vi "CRISPR Program.vi"() -> ()   [LabVIEW 2024]
uses:
  States Enum.ctl
panel:
  in  "Splice 1: Base Pair to be used":enum16{"T-A", "A-T", "C-G", "G-C"}(ring)
  in  "Splice 1: Base Pair No.  in Codon":dbl=1.0 min=1.0 max=3.0
  in  "Splice 1: Codon No.":dbl=1.0 min=1.0 max=5.0
  out "% of C-G(G-C) in Modified DNA Sequence":dbl format="%#.0f"
  out "% of A-T(T-A) in Modified DNA Sequence":dbl format="%#.0f"
  out "Modified DNA A-COUNT":i32
  out "Modified DNA C-COUNT":i32
  out "Modified DNA G-COUNT":i32
  out "Modified DNA T-COUNT":i32
  in  "Stop":bool
  out "Modified DNA Sequence":string[][](array[string])
  in  "Splice":bool
  in  "DNA Splice Selector":T1(ring)=enum."Splice 2"
  out "% of C-G(G-C) in DNA Sequence":dbl format="%#.0f"
  out "% of A-T(T-A) in DNA Sequence":dbl format="%#.0f"
  out "DNA A-COUNT":i32
  out "DNA C-COUNT":i32
  out "DNA G-COUNT":i32
  out "DNA T-COUNT":i32
  out "DNA Sequence":string[][](array[string])
  out "RNA Sequence with Mutation Genes Removed":string[][](array[string])
  out "error out":errorcluster
  in  "error in (no error)":errorcluster
  out "Original RNA Sequence":string[][](array[string])
  # "Normal DNA Sequence"
  # "Modified DNA Sequence"
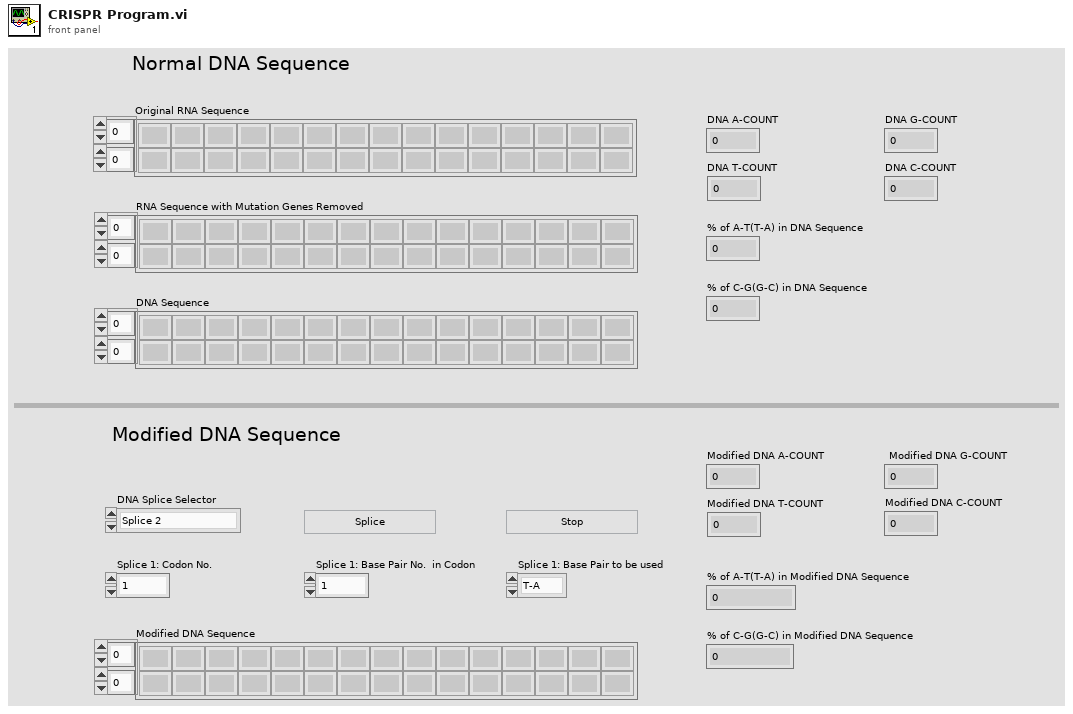
[diagram p1: front panel]
types:
  T1 = enum16{"Splice 1", "Splice 2", "Splice 3", "Splice 4", "No Splice"}
  T2 = typedef "States Enum.ctl" = enum16{"Remove Mutation", "Initialize", "DNA Sequence", "DNA Result", "Modified DNA Sequence", "Modified DNA Result", "Wait"}
  T3 = enum8{"Enabled", "Disabled", "Disabled and Grayed Out"}
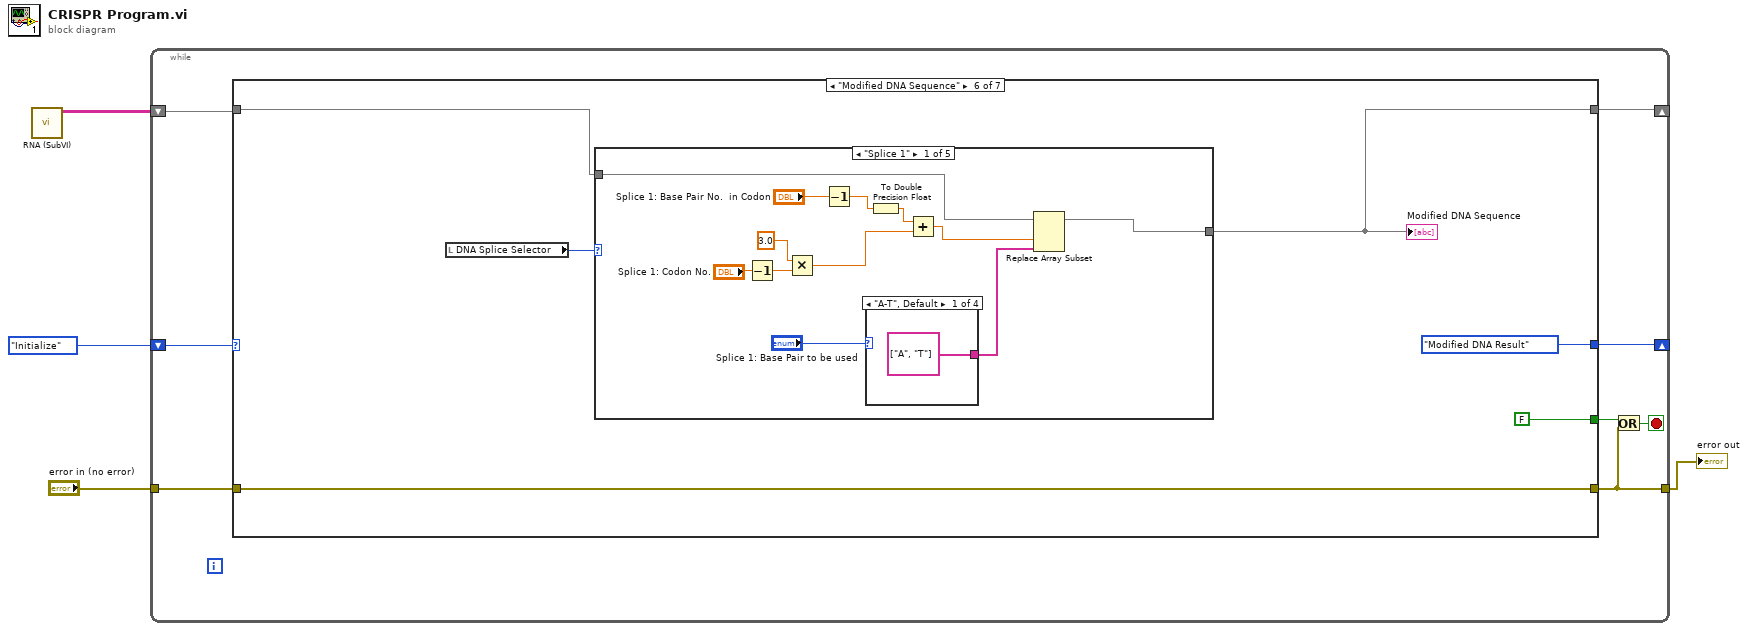
[diagram p0: block diagram]
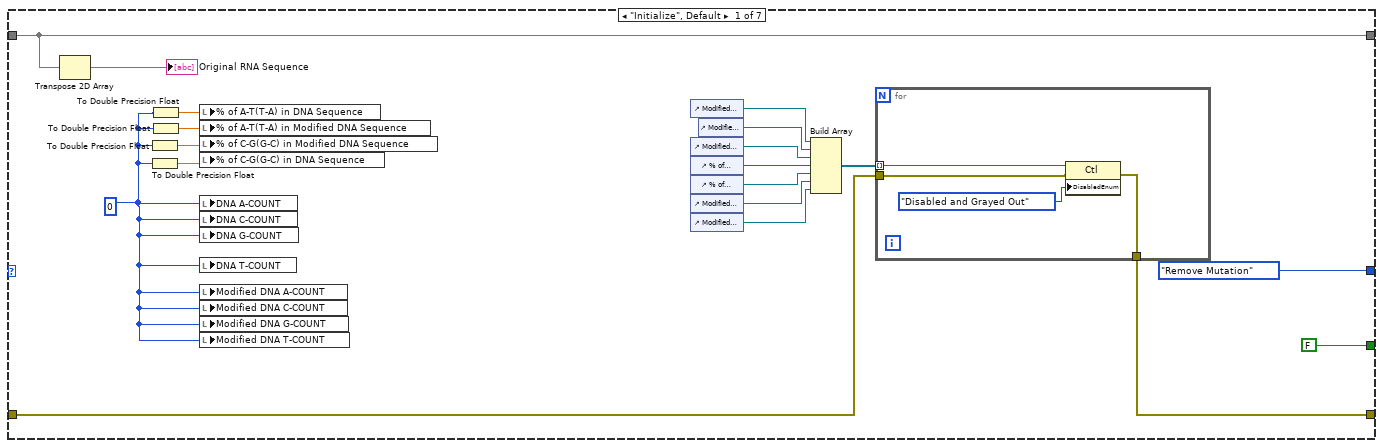
[diagram p2: hidden frame]
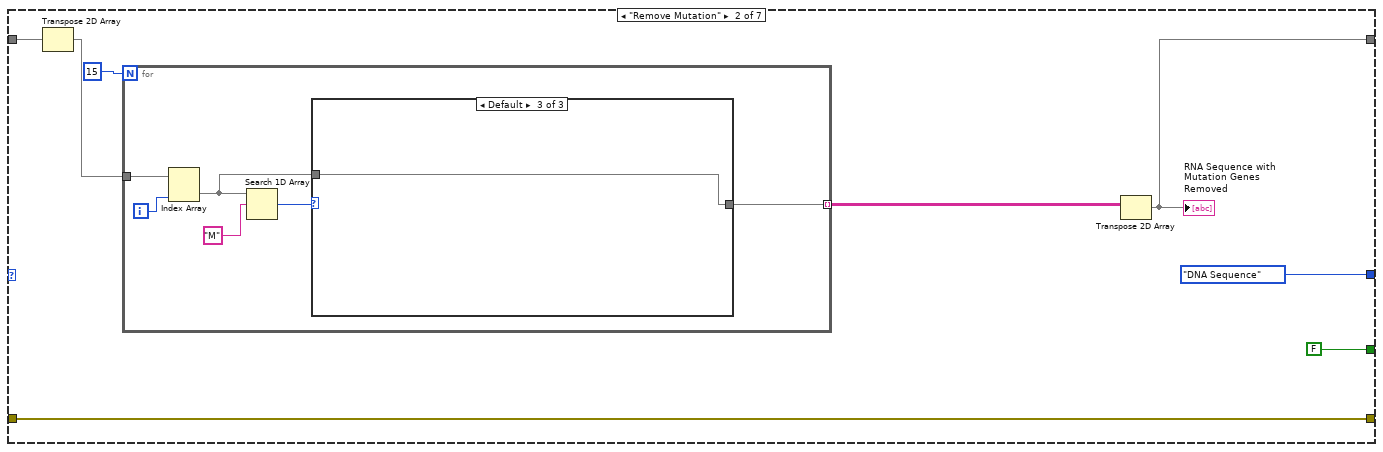
[diagram p3: hidden frame]
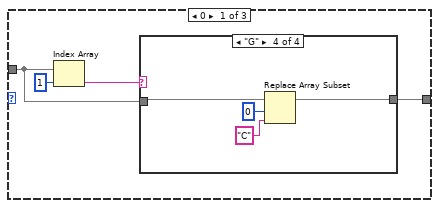
[diagram p4: hidden frame]
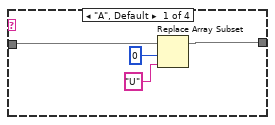
[diagram p5: hidden frame]
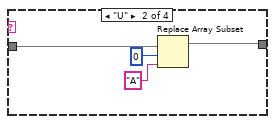
[diagram p6: hidden frame]
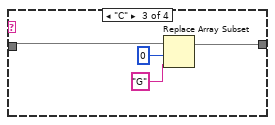
[diagram p7: hidden frame]
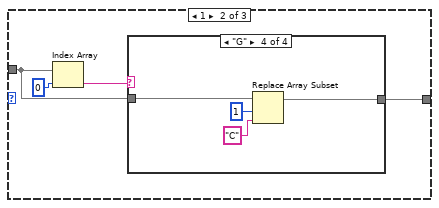
[diagram p8: hidden frame]
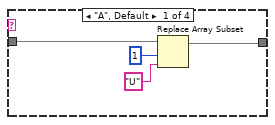
[diagram p9: hidden frame]
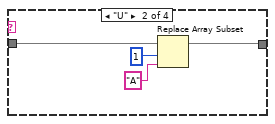
[diagram p10: hidden frame]
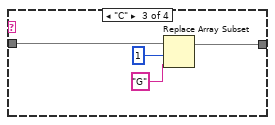
[diagram p11: hidden frame]
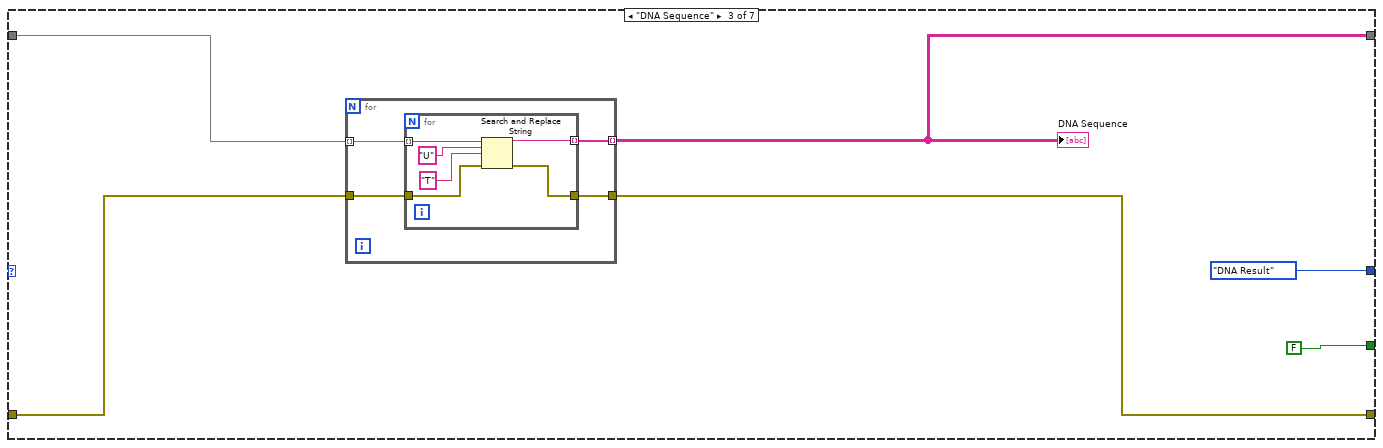
[diagram p12: hidden frame]
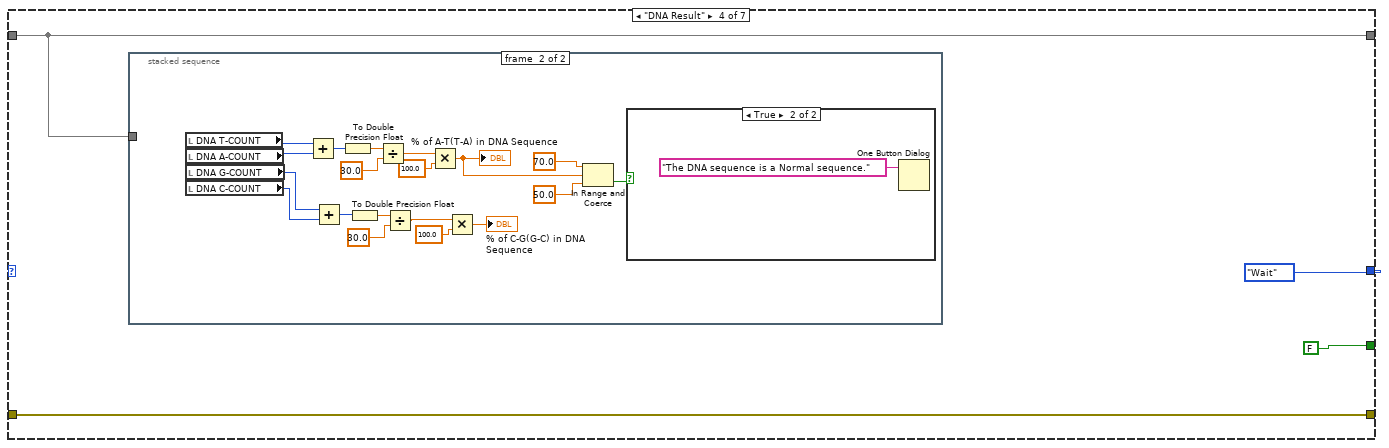
[diagram p13: hidden frame]
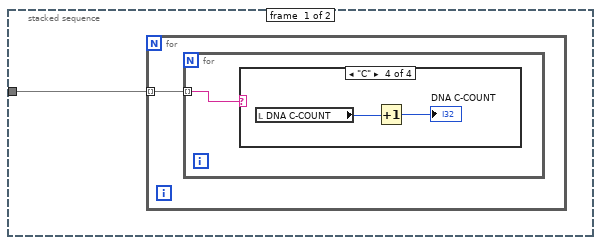
[diagram p14: hidden frame]
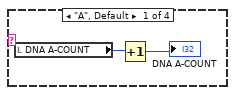
[diagram p15: hidden frame]
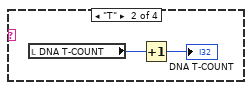
[diagram p16: hidden frame]
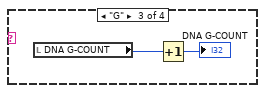
[diagram p17: hidden frame]
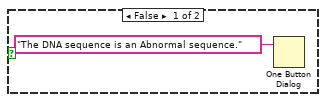
[diagram p18: hidden frame]
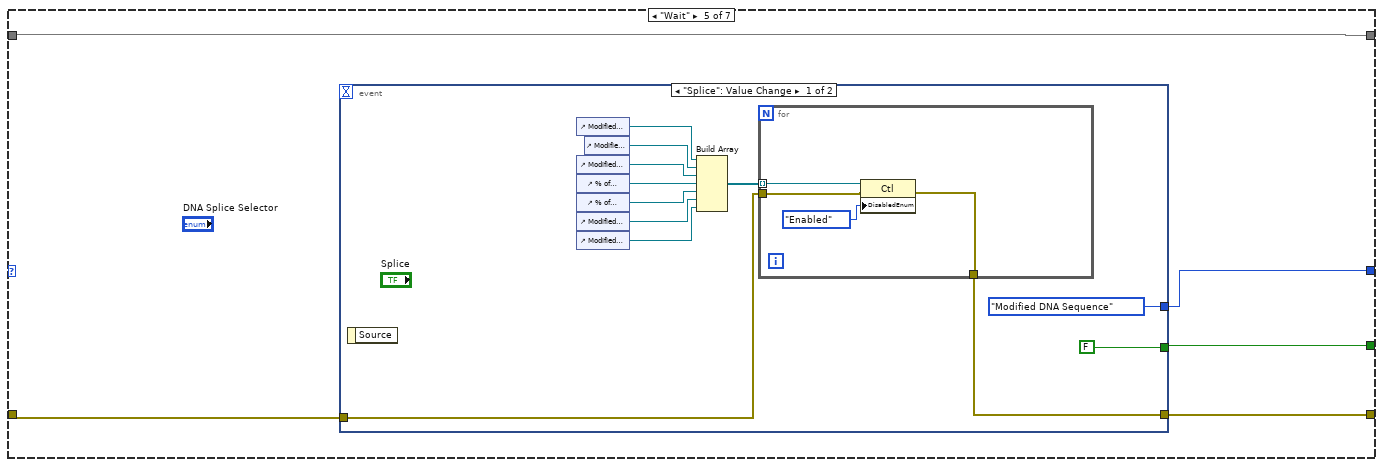
[diagram p19: hidden frame]
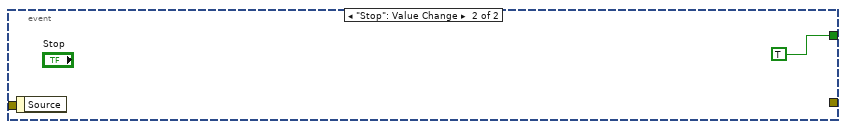
[diagram p20: hidden frame]
diagram:
  n1 = call "RNA (SubVI).vi"() -> ("RNA Sequence"=w2:string[][])  [unwired: 11 in]
  n2 = while {
    shift-right: [w5] -> _
    shift-left: States_Enum."Initialize" -> [w6]
    shift-right: [w11] -> _
    shift-left: w2 -> [w12]
    tunnel: "error in (no error)" -> [w10]
    tunnel: [w7] -> w3
    stop <- w9 stop-if-true
    n3 = case shown="\"Modified DNA Sequence\"" w6 {
      tunnel: w12 -> [w30 w43 w96 w109 w147 w167 w217]
      tunnel: [w30 w37 w95 w109 w147 w165 w217] -> w11
      tunnel: [States_Enum."Remove Mutation" States_Enum."DNA Sequence" States_Enum."DNA Result" States_Enum."Wait" w145 States_Enum."Modified DNA Result" States_Enum."Initialize"] -> w5
      tunnel: w10 -> [w14 w41 w93 w110 w146 w170 w218]
      tunnel: [w13 w41 w92 w110 w143 w170 w218] -> w7
      tunnel: [FALSE FALSE FALSE FALSE w144 FALSE TRUE] -> w8
      frame "Initialize", Default {
        w23 = 0 ("DNA A-COUNT")
        n4 = Transpose 2D Array(2D array=w30) -> (transposed array=→"Original RNA Sequence":string[][])
        n5 = To Double Precision Float(number=w23) -> (double precision float=w25:dbl)
        n6 = To Double Precision Float(number=w23) -> (double precision float=w24:dbl)
        n7 = To Double Precision Float(number=w23) -> (double precision float=w27:dbl)
        n8 = To Double Precision Float(number=w23) -> (double precision float=w26:dbl)
        n9 = local write "% of A-T(T-A) in DNA Sequence"(w27) -> ()
        n10 = local write "% of A-T(T-A) in Modified DNA Sequence"(w26) -> ()
        n11 = local write "% of C-G(G-C) in Modified DNA Sequence"(w25) -> ()
        n12 = local write "% of C-G(G-C) in DNA Sequence"(w24) -> ()
        n13 = local write "DNA A-COUNT"(w23) -> ()
        n14 = local write "DNA C-COUNT"(w23) -> ()
        n15 = local write "DNA G-COUNT"(w23) -> ()
        n16 = local write "DNA T-COUNT"(w23) -> ()
        n17 = local write "Modified DNA A-COUNT"(w23) -> ()
        n18 = local write "Modified DNA C-COUNT"(w23) -> ()
        n19 = local write "Modified DNA G-COUNT"(w23) -> ()
        n20 = local write "Modified DNA T-COUNT"(w23) -> ()
        n21 = control-ref of="Modified DNA C-COUNT"() -> (w22:refnum<vi>)
        n22 = control-ref of="Modified DNA A-COUNT"() -> (w20:refnum<vi>)
        n23 = control-ref of="% of C-G(G-C) in Modified DNA Sequence"() -> (w19:refnum<vi>)
        n24 = control-ref of="% of A-T(T-A) in Modified DNA Sequence"() -> (w18:refnum<vi>)
        n25 = control-ref of="Modified DNA T-COUNT"() -> (w17:refnum<vi>)
        n26 = control-ref of="Modified DNA G-COUNT"() -> (w16:refnum<vi>)
        n27 = control-ref of="Modified DNA Sequence"() -> (w21:refnum<vi>)
        n28 = Build Array(w22, w21, w20, w19, w18, w17, w16) -> (w15:refnum<vi>[])
        n29 = for {
          tunnel: w15 -> [w35] mode=indexing
          tunnel: w14 -> [w33]
          tunnel: [w32] -> w13
          n30 = property class="Ctl"(reference=w35, error in=w33, "DisabledEnum"=T3."Disabled and Grayed Out" ("Disabled")) -> (error out=w32:errorcluster)  [unwired: 1 out]
        }
      }
      frame "Remove Mutation" {
        n31 = Transpose 2D Array(2D array=w43) -> (transposed array=w39:string[][])
        n32 = for {
          N: 15 -> [_]
          tunnel: [w47] -> w38 mode=indexing
          tunnel: w39 -> [w46]
          i -> [w49]
          n33 = Index Array(array=w46, index (col)=w49) -> (element=w45:string[])  [unwired: 1 in]
          n34 = Search 1D Array(1D array=w45, element="M") -> (index of element=w48:i32)  [unwired: 1 in]
          n35 = case shown="Default" w48 {
            tunnel: w45 -> [w51 w71 w90]
            tunnel: [w52 w72 w90] -> w47
            frame 0 {
              n36 = Index Array(array=w51, index=1) -> (element=w50:string)
              n37 = case shown="\"G\"" w50 {
                tunnel: w51 -> [w54 w58 w62 w66]
                tunnel: [w55 w59 w63 w67] -> w52
                frame "A", Default {
                  n38 = Replace Array Subset(array=w54, new element="U" ("element"), index=0) -> (w55:string[])
                }
                frame "U" {
                  n39 = Replace Array Subset(array=w58, new element="A" ("element"), index=0) -> (w59:string[])
                }
                frame "C" {
                  n40 = Replace Array Subset(array=w62, new element="G" ("element"), index=0) -> (w63:string[])
                }
                frame "G" {
                  n41 = Replace Array Subset(array=w66, new element="C" ("element"), index=0) -> (w67:string[])
                }
              }
            }
            frame 1 {
              n42 = Index Array(array=w71, index=0) -> (element=w70:string)
              n43 = case shown="\"G\"" w70 {
                tunnel: w71 -> [w74 w78 w82 w86]
                tunnel: [w75 w79 w83 w87] -> w72
                frame "A", Default {
                  n44 = Replace Array Subset(array=w74, new element="U" ("element"), index=1) -> (w75:string[])
                }
                frame "U" {
                  n45 = Replace Array Subset(array=w78, new element="A" ("element"), index=1) -> (w79:string[])
                }
                frame "C" {
                  n46 = Replace Array Subset(array=w82, new element="G" ("element"), index=1) -> (w83:string[])
                }
                frame "G" {
                  n47 = Replace Array Subset(array=w86, new element="C" ("element"), index=1) -> (w87:string[])
                }
              }
            }
            frame Default {
            }
          }
        }
        n48 = Transpose 2D Array(2D array=w38) -> (transposed array=w37:string[][])
        "RNA Sequence with Mutation Genes Removed" <- w37
      }
      frame "DNA Sequence" {
        n49 = for {
          tunnel: w96 -> [w100] mode=indexing
          tunnel: [w99] -> w95 mode=indexing
          tunnel: w93 -> [w98]
          tunnel: [w97] -> w92
          n50 = for {
            tunnel: w100 -> [w106] mode=indexing
            tunnel: [w105] -> w99 mode=indexing
            tunnel: w98 -> [w102]
            tunnel: [w101] -> w97
            n51 = Search and Replace String(input string=w106, search string="U", replace string="T" ("replace string (\"\")"), error in=w102) -> (result string=w105:string, error out=w101:errorcluster)  [unwired: 4 in, 2 out]
          }
        }
        "DNA Sequence" <- w95
      }
      frame "DNA Result" {
        n52 = stacked-sequence {
          tunnel: w109 -> [w111 _]
          frame #0 {
            n53 = for {
              tunnel: w111 -> [w112] mode=indexing
              n54 = for {
                tunnel: w112 -> [w113] mode=indexing
                n55 = case shown="\"C\"" w113 {
                  frame "A", Default {
                    n56 = local read "DNA A-COUNT"() -> (w115:i32)
                    n57 = Increment(x=w115) -> (x+1=→"DNA A-COUNT":i32)
                  }
                  frame "T" {
                    n58 = local read "DNA T-COUNT"() -> (w117:i32)
                    n59 = Increment(x=w117) -> (x+1=→"DNA T-COUNT":i32)
                  }
                  frame "G" {
                    n60 = local read "DNA G-COUNT"() -> (w119:i32)
                    n61 = Increment(x=w119) -> (x+1=→"DNA G-COUNT":i32)
                  }
                  frame "C" {
                    n62 = local read "DNA C-COUNT"() -> (w121:i32)
                    n63 = Increment(x=w121) -> (x+1=→"DNA C-COUNT":i32)
                  }
                }
              }
            }
          }
          frame #1 {
            n64 = local read "DNA T-COUNT"() -> (w140:i32)
            n65 = local read "DNA A-COUNT"() -> (w139:i32)
            n66 = local read "DNA G-COUNT"() -> (w137:i32)
            n67 = local read "DNA C-COUNT"() -> (w138:i32)
            n68 = Add(x=w140, y=w139) -> (x+y=w136:i32)
            n69 = Add(x=w137, y=w138) -> (x+y=w131:i32)
            n70 = To Double Precision Float(number=w136) -> (double precision float=w134:dbl)
            n71 = To Double Precision Float(number=w131) -> (double precision float=w133:dbl)
            n72 = Divide(x=w134, y=30.0) -> (x/y=w130:dbl)
            n73 = Divide(x=w133, y=30.0) -> (x/y=w127:dbl)
            n74 = Multiply(x=w130, y=100.0) -> (x*y=w122:dbl)
            "% of A-T(T-A) in DNA Sequence" <- w122
            n75 = Multiply(x=w127, y=100.0) -> (x*y=→"% of C-G(G-C) in DNA Sequence":dbl)
            n76 = In Range and Coerce(upper limit=70.0, x=w122, lower limit=50.0) -> (In Range?=w123:bool)  [unwired: 1 out]
            n77 = case shown="True" w123 {
              frame False {
                n78 = One Button Dialog(message="The DNA sequence is an Abnormal sequence.") -> ()  [unwired: 1 in, 1 out]
              }
              frame True {
                n79 = One Button Dialog(message="The DNA sequence is a Normal sequence.") -> ()  [unwired: 1 in, 1 out]
              }
            }
          }
        }
      }
      frame "Wait" {
        n80 = event shown="[0] \"Splice\": Value Change" {
          selector: _ -> [_ _]
          dyn-events: _ -> [_ _]
          timeout: _ -> [_ _]
          tunnel: w146 -> [w149 _]
          tunnel: [States_Enum."Modified DNA Sequence" _] -> w145
          tunnel: [FALSE TRUE] -> w144
          tunnel: [w148 _] -> w143
          event "Splice": Value Change {
            n81 = event-data() -> ()  [unwired: 1 in, 1 out]
            n82 = control-ref of="Modified DNA C-COUNT"() -> (w157:refnum<vi>)
            n83 = control-ref of="Modified DNA A-COUNT"() -> (w155:refnum<vi>)
            n84 = control-ref of="% of C-G(G-C) in Modified DNA Sequence"() -> (w154:refnum<vi>)
            n85 = control-ref of="% of A-T(T-A) in Modified DNA Sequence"() -> (w153:refnum<vi>)
            n86 = control-ref of="Modified DNA T-COUNT"() -> (w152:refnum<vi>)
            n87 = control-ref of="Modified DNA G-COUNT"() -> (w151:refnum<vi>)
            n88 = control-ref of="Modified DNA Sequence"() -> (w156:refnum<vi>)
            n89 = Build Array(w157, w156, w155, w154, w153, w152, w151) -> (w150:refnum<vi>[])
            n90 = for {
              tunnel: w150 -> [w163] mode=indexing
              tunnel: w149 -> [w161]
              tunnel: [w160] -> w148
              n91 = property class="Ctl"(reference=w163, error in=w161, "DisabledEnum"=T3."Enabled" ("Disabled")) -> (error out=w160:errorcluster)  [unwired: 1 out]
            }
          }
          event "Stop": Value Change {
            n92 = event-data() -> ()  [unwired: 1 in, 1 out]
          }
        }
      }
      frame "Modified DNA Sequence" {
        n93 = local read "DNA Splice Selector"() -> (w168:T1)
        n94 = case shown="\"Splice 1\"" w168 {
          tunnel: w167 -> [w180 w191 w194 w204 w214]
          tunnel: [w175 w187 w192 w203 w214] -> w165
          frame "Splice 1" {
            n95 = Decrement(x="Splice 1: Codon No.") -> (x-1=w181:dbl)
            n96 = Multiply(x=3.0, y=w181) -> (x*y=w179:dbl)
            n97 = Decrement(x="Splice 1: Base Pair No.  in Codon") -> (x-1=w178:dbl)
            n98 = case shown="\"A-T\", Default" "Splice 1: Base Pair to be used" {
              tunnel: [string[] ["A", "T"] string[] ["T", "A"] string[] ["G", "C"] string[] ["C", "G"]] -> w176
              frame "A-T", Default {
              }
              frame "T-A" {
              }
              frame "G-C" {
              }
              frame "C-G" {
              }
            }
            n99 = To Double Precision Float(number=w178) -> (double precision float=w174:dbl)
            n100 = Add(x=w174, y=w179) -> (x+y=w177:dbl)
            n101 = Replace Array Subset(array=w180, new element=w176, index (col)=w177) -> (w175:string[][])  [unwired: 1 in]
          }
          frame "Splice 2" {
            n102 = Replace Array Subset(array=w191, new element=string[][] [["T", "G", "C"], ["A", "C", "G"]], index (row)=0, index (col)=3) -> (w187:string[][])
          }
          frame "Splice 3" {
            n103 = flat-sequence {
              tunnel: w194 -> [w198]
              tunnel: [w195] -> w193
              tunnel: w193 -> [w200]
              tunnel: [w199] -> w192
              frame #0 {
                n104 = Replace Array Subset(array=w198, new element=string[] ["T", "A"] ("new element/subarray"), index (col)=7) -> (w195:string[][])  [unwired: 1 in]
              }
              frame #1 {
                n105 = Replace Array Subset(array=w200, new element=string[] ["A", "T"] ("new element/subarray"), index (col)=9) -> (w199:string[][])  [unwired: 1 in]
              }
            }
          }
          frame "Splice 4" {
            n106 = for {
              N: 5 -> [_]
              shift-right: [w207] -> w203
              shift-left: w204 -> [w208]
              i -> [w211]
              n107 = Multiply(x=2, y=w211) -> (x*y=w212:i32)
              n108 = Add(x=w212, y=w211) -> (x+y=w209:i32)
              n109 = Replace Array Subset(array=w208, new element=string[] ["A", "T"] ("new element/subarray"), index (col)=w209) -> (w207:string[][])  [unwired: 1 in]
              n110 = Wait (ms)(milliseconds to wait=u32 1000) -> ()  [unwired: 1 out]
            }
          }
          frame "No Splice", Default {
          }
        }
        "Modified DNA Sequence" <- w165
      }
      frame "Modified DNA Result" {
        n111 = stacked-sequence {
          tunnel: w217 -> [w219 _]
          frame #0 {
            n112 = for {
              tunnel: w219 -> [w220] mode=indexing
              n113 = for {
                tunnel: w220 -> [w221] mode=indexing
                n114 = case shown="\"C\"" w221 {
                  frame "A", Default {
                    n115 = local read "Modified DNA A-COUNT"() -> (w223:i32)
                    n116 = Increment(x=w223) -> (x+1=→"Modified DNA A-COUNT":i32)
                  }
                  frame "T" {
                    n117 = local read "Modified DNA T-COUNT"() -> (w225:i32)
                    n118 = Increment(x=w225) -> (x+1=→"Modified DNA T-COUNT":i32)
                  }
                  frame "G" {
                    n119 = local read "Modified DNA G-COUNT"() -> (w227:i32)
                    n120 = Increment(x=w227) -> (x+1=→"Modified DNA G-COUNT":i32)
                  }
                  frame "C" {
                    n121 = local read "Modified DNA C-COUNT"() -> (w229:i32)
                    n122 = Increment(x=w229) -> (x+1=→"Modified DNA C-COUNT":i32)
                  }
                }
              }
            }
          }
          frame #1 {
            n123 = local read "Modified DNA G-COUNT"() -> (w245:i32)
            n124 = local read "Modified DNA C-COUNT"() -> (w246:i32)
            n125 = local read "Modified DNA T-COUNT"() -> (w247:i32)
            n126 = local read "Modified DNA A-COUNT"() -> (w248:i32)
            n127 = Add(x=w248, y=w247) -> (x+y=w244:i32)
            n128 = Add(x=w245, y=w246) -> (x+y=w239:i32)
            n129 = To Double Precision Float(number=w244) -> (double precision float=w242:dbl)
            n130 = To Double Precision Float(number=w239) -> (double precision float=w241:dbl)
            n131 = Divide(x=w242, y=30.0) -> (x/y=w238:dbl)
            n132 = Divide(x=w241, y=30.0) -> (x/y=w235:dbl)
            n133 = Multiply(x=w238, y=100.0) -> (x*y=w230:dbl)
            "% of A-T(T-A) in Modified DNA Sequence" <- w230
            n134 = Multiply(x=w235, y=100.0) -> (x*y=→"% of C-G(G-C) in Modified DNA Sequence":dbl)
            n135 = In Range and Coerce(upper limit=70.0, x=w230, lower limit=50.0) -> (In Range?=w232:bool)  [unwired: 1 out]
            n136 = case shown="False" w232 {
              frame False {
                n137 = One Button Dialog(message="The Modified DNA sequence is an Abnormal sequence.", button name ("OK")="Ok") -> ()  [unwired: 1 out]
              }
              frame True {
                n138 = One Button Dialog(message="The  Modified DNA sequence is a Normal sequence.") -> ()  [unwired: 1 in, 1 out]
              }
            }
          }
        }
      }
    }
    n139 = Or(x=w8, y=w7) -> (x .or. y?=w9:bool)
  }
  "error out" <- w3
